vi "WaitForEdge.fpga.vi"(10 "x (in)":u16) -> ()   [LabVIEW 2012]
uses:
  <vilib>/rvi/eio/common/nirviEmuTemplateMethod_errors.vi
  <vilib>/eio/EIONode/EIONode.xnode
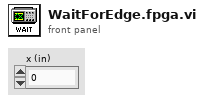
[diagram p1: front panel]
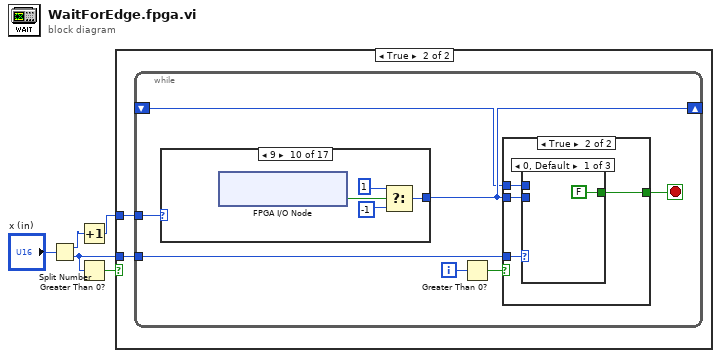
[diagram p0: block diagram]
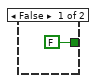
[diagram p3: hidden frame]
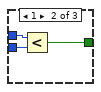
[diagram p4: hidden frame]
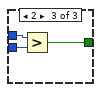
[diagram p5: hidden frame]
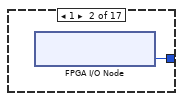
[diagram p7: hidden frame]
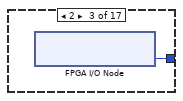
[diagram p8: hidden frame]
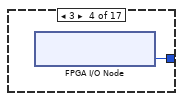
[diagram p9: hidden frame]
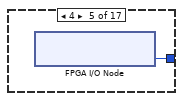
[diagram p10: hidden frame]
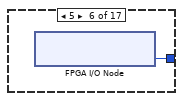
[diagram p11: hidden frame]
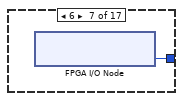
[diagram p12: hidden frame]
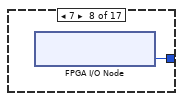
[diagram p13: hidden frame]
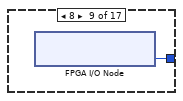
[diagram p14: hidden frame]
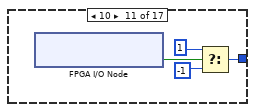
[diagram p15: hidden frame]
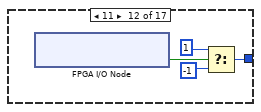
[diagram p16: hidden frame]
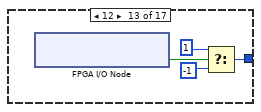
[diagram p17: hidden frame]
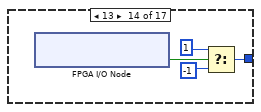
[diagram p18: hidden frame]
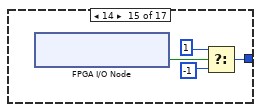
[diagram p19: hidden frame]
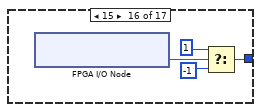
[diagram p20: hidden frame]
diagram:
  n1 = Split Number(x="x (in)") -> (hi(x)=w2:u8, lo(x)=w3:u8)
  n2 = Increment(x=w2) -> (x+1=w1:u8)
  n3 = Greater Than 0?(x=w3) -> (x > 0?=w4:bool)
  n4 = case shown="True" w4 {
    tunnel: w1 -> [_ w7]
    tunnel: w3 -> [_ w6]
    frame False {
    }
    frame True {
      n5 = while {
        tunnel: w7 -> [w14]
        tunnel: w6 -> [w13]
        shift-right: [w12] -> _
        shift-left: _ -> [w11]
        i -> [w10]
        stop <- w8 stop-if-true
        n6 = case shown="9" w14 {
          tunnel: [_ w27 w28 w29 w30 w31 w32 w33 w34 w36 w40 w44 w50 w52 w56 w60 w64] -> w12
          frame 0, Default {
          }
          frame 1 {
            n7 = xnode "FPGA I/O Node"() -> ("Connector0/AI0"=w27:i16)  [unwired: 1 in, 1 out]
          }
          frame 2 {
            n8 = xnode "FPGA I/O Node"() -> ("Connector0/AI1"=w28:i16)  [unwired: 1 in, 1 out]
          }
          frame 3 {
            n9 = xnode "FPGA I/O Node"() -> ("Connector0/AI2"=w29:i16)  [unwired: 1 in, 1 out]
          }
          frame 4 {
            n10 = xnode "FPGA I/O Node"() -> ("Connector0/AI3"=w30:i16)  [unwired: 1 in, 1 out]
          }
          frame 5 {
            n11 = xnode "FPGA I/O Node"() -> ("Connector0/AI4"=w31:i16)  [unwired: 1 in, 1 out]
          }
          frame 6 {
            n12 = xnode "FPGA I/O Node"() -> ("Connector0/AI5"=w32:i16)  [unwired: 1 in, 1 out]
          }
          frame 7 {
            n13 = xnode "FPGA I/O Node"() -> ("Connector0/AI6"=w33:i16)  [unwired: 1 in, 1 out]
          }
          frame 8 {
            n14 = xnode "FPGA I/O Node"() -> ("Connector0/AI7"=w34:i16)  [unwired: 1 in, 1 out]
          }
          frame 9 {
            n15 = xnode "FPGA I/O Node"() -> ("Connector0/DIO8"=w35:bool)  [unwired: 1 in, 1 out]
            n16 = Select(t=i16 1, s=w35, f=i16 -1 ("t")) -> (s? t:f=w36:i16)
          }
          frame 10 {
            n17 = xnode "FPGA I/O Node"() -> ("Connector0/DIO9"=w39:bool)  [unwired: 1 in, 1 out]
            n18 = Select(t=i16 1, s=w39, f=i16 -1 ("t")) -> (s? t:f=w40:i16)
          }
          frame 11 {
            n19 = xnode "FPGA I/O Node"() -> ("Connector0/DIO10"=w43:bool)  [unwired: 1 in, 1 out]
            n20 = Select(t=i16 1, s=w43, f=i16 -1 ("t")) -> (s? t:f=w44:i16)
          }
          frame 12 {
            n21 = xnode "FPGA I/O Node"() -> ("Connector0/DIO11"=w49:bool)  [unwired: 1 in, 1 out]
            n22 = Select(t=i16 1, s=w49, f=i16 -1 ("t")) -> (s? t:f=w50:i16)
          }
          frame 13 {
            n23 = xnode "FPGA I/O Node"() -> ("Connector0/DIO12"=w51:bool)  [unwired: 1 in, 1 out]
            n24 = Select(t=i16 1, s=w51, f=i16 -1 ("t")) -> (s? t:f=w52:i16)
          }
          frame 14 {
            n25 = xnode "FPGA I/O Node"() -> ("Connector0/DIO13"=w55:bool)  [unwired: 1 in, 1 out]
            n26 = Select(t=i16 1, s=w55, f=i16 -1 ("t")) -> (s? t:f=w56:i16)
          }
          frame 15 {
            n27 = xnode "FPGA I/O Node"() -> ("Connector0/DIO14"=w59:bool)  [unwired: 1 in, 1 out]
            n28 = Select(t=i16 1, s=w59, f=i16 -1 ("t")) -> (s? t:f=w60:i16)
          }
          frame 16 {
            n29 = xnode "FPGA I/O Node"() -> ("Connector0/DIO15"=w63:bool)  [unwired: 1 in, 1 out]
            n30 = Select(t=i16 1, s=w63, f=i16 -1 ("t")) -> (s? t:f=w64:i16)
          }
        }
        n31 = Greater Than 0?(x=w10) -> (x > 0?=w9:bool)
        n32 = case shown="True" w9 {
          tunnel: w13 -> [_ w19]
          tunnel: w12 -> [_ w18]
          tunnel: w11 -> [_ w17]
          tunnel: [FALSE w16] -> w8
          frame False {
          }
          frame True {
            n33 = case shown="0, Default" w19 {
              tunnel: w18 -> [_ w22 w25]
              tunnel: w17 -> [_ w23 w26]
              tunnel: [FALSE w21 w24] -> w16
              frame 0, Default {
              }
              frame 1 {
                n34 = Less?(x=w23, y=w22) -> (x < y?=w21:bool)
              }
              frame 2 {
                n35 = Greater?(x=w26, y=w25) -> (0:w24:bool)
              }
            }
          }
        }
      }
    }
  }
